vi "borders and shading constant (table).vi"() -> (0 "borders and shading":T1={"OutsideLineStyle"=1, "OutsideColor"=-16777216, "OutsideLineWidth"=2, "InsideLineStyle"=1, "InsideColor"=-16777216, "InsideLineWidth"=2, "BackgroundPatternColor"=-16777216} {"InsideLineStyle" items=["wdLineStyleNone", "wdLineStyleSingle", "wdLineStyleDot", "wdLineStyleDashSmallGap", "wdLineStyleDashLargeGap", "wdLineStyleDashDot", "wdLineStyleDashDotDot", "wdLineStyleDouble", "wdLineStyleTriple", "wdLineStyleThinThickSmallGap", "wdLineStyleThickThinSmallGap", "wdLineStyleThinThickThinSmallGap", "wdLineStyleThinThickMedGap", "wdLineStyleThickThinMedGap", "wdLineStyleThinThickThinMedGap", "wdLineStyleThinThickLargeGap", "wdLineStyleThickThinLargeGap", "wdLineStyleThinThickThinLargeGap", "wdLineStyleSingleWavy", "wdLineStyleDoubleWavy", "wdLineStyleDashDotStroked", "wdLineStyleEmboss3D", "wdLineStyleEngrave3D", "wdLineStyleOutset", "wdLineStyleInset"]; "BackgroundPatternColor" items=["wdColorAutomatic"=-16777216, "wdColorBlack"=0, "wdColorBlue"=16711680, "wdColorTurquoise"=16776960, "wdColorBrightGreen"=65280, "wdColorPink"=16711935, "wdColorRed"=255, "wdColorYellow"=65535, "wdColorWhite"=16777215, "wdColorDarkBlue"=8388608, "wdColorTeal"=8421376, "wdColorGreen"=32768, "wdColorViolet"=8388736, "wdColorDarkRed"=128, "wdColorDarkYellow"=32896, "wdColorBrown"=13209, "wdColorOliveGreen"=13107, "wdColorDarkGreen"=13056, "wdColorDarkTeal"=6697728, "wdColorIndigo"=10040115, "wdColorOrange"=26367, "wdColorBlueGray"=10053222, "wdColorLightOrange"=39423, "wdColorLime"=52377, "wdColorSeaGreen"=6723891, "wdColorAqua"=13421619, "wdColorLightBlue"=16737843, "wdColorGold"=52479, "wdColorSkyBlue"=16763904, "wdColorPlum"=6697881, "wdColorRose"=13408767, "wdColorTan"=10079487, "wdColorLightYellow"=10092543, "wdColorLightGreen"=13434828, "wdColorLightTurquoise"=16777164, "wdColorPaleBlue"=16764057, "wdColorLavender"=16751052, "wdColorGray05"=15987699, "wdColorGray10"=15132390, "wdColorGray125"=14737632, "wdColorGray15"=14277081, "wdColorGray20"=13421772, "wdColorGray25"=12632256, "wdColorGray30"=11776947, "wdColorGray35"=10921638, "wdColorGray375"=10526880, "wdColorGray40"=10066329, "wdColorGray45"=9211020, "wdColorGray50"=8421504, "wdColorGray55"=7566195, "wdColorGray60"=6710886, "wdColorGray625"=6316128, "wdColorGray65"=5855577, "wdColorGray70"=5000268, "wdColorGray75"=4210752, "wdColorGray80"=3355443, "wdColorGray85"=2500134, "wdColorGray875"=2105376, "wdColorGray90"=1644825, "wdColorGray95"=789516]; "InsideLineWidth" items=["wdLineWidth025pt"=2, "wdLineWidth050pt"=4, "wdLineWidth075pt"=6, "wdLineWidth100pt"=8, "wdLineWidth150pt"=12, "wdLineWidth225pt"=18, "wdLineWidth300pt"=24, "wdLineWidth450pt"=36, "wdLineWidth600pt"=48]; "InsideColor" items=["wdColorAutomatic"=-16777216, "wdColorBlack"=0, "wdColorBlue"=16711680, "wdColorTurquoise"=16776960, "wdColorBrightGreen"=65280, "wdColorPink"=16711935, "wdColorRed"=255, "wdColorYellow"=65535, "wdColorWhite"=16777215, "wdColorDarkBlue"=8388608, "wdColorTeal"=8421376, "wdColorGreen"=32768, "wdColorViolet"=8388736, "wdColorDarkRed"=128, "wdColorDarkYellow"=32896, "wdColorBrown"=13209, "wdColorOliveGreen"=13107, "wdColorDarkGreen"=13056, "wdColorDarkTeal"=6697728, "wdColorIndigo"=10040115, "wdColorOrange"=26367, "wdColorBlueGray"=10053222, "wdColorLightOrange"=39423, "wdColorLime"=52377, "wdColorSeaGreen"=6723891, "wdColorAqua"=13421619, "wdColorLightBlue"=16737843, "wdColorGold"=52479, "wdColorSkyBlue"=16763904, "wdColorPlum"=6697881, "wdColorRose"=13408767, "wdColorTan"=10079487, "wdColorLightYellow"=10092543, "wdColorLightGreen"=13434828, "wdColorLightTurquoise"=16777164, "wdColorPaleBlue"=16764057, "wdColorLavender"=16751052, "wdColorGray05"=15987699, "wdColorGray10"=15132390, "wdColorGray125"=14737632, "wdColorGray15"=14277081, "wdColorGray20"=13421772, "wdColorGray25"=12632256, "wdColorGray30"=11776947, "wdColorGray35"=10921638, "wdColorGray375"=10526880, "wdColorGray40"=10066329, "wdColorGray45"=9211020, "wdColorGray50"=8421504, "wdColorGray55"=7566195, "wdColorGray60"=6710886, "wdColorGray625"=6316128, "wdColorGray65"=5855577, "wdColorGray70"=5000268, "wdColorGray75"=4210752, "wdColorGray80"=3355443, "wdColorGray85"=2500134, "wdColorGray875"=2105376, "wdColorGray90"=1644825, "wdColorGray95"=789516]; "OutsideLineWidth" items=["wdLineWidth025pt"=2, "wdLineWidth050pt"=4, "wdLineWidth075pt"=6, "wdLineWidth100pt"=8, "wdLineWidth150pt"=12, "wdLineWidth225pt"=18, "wdLineWidth300pt"=24, "wdLineWidth450pt"=36, "wdLineWidth600pt"=48]; "OutsideColor" items=["wdColorAutomatic"=-16777216, "wdColorBlack"=0, "wdColorBlue"=16711680, "wdColorTurquoise"=16776960, "wdColorBrightGreen"=65280, "wdColorPink"=16711935, "wdColorRed"=255, "wdColorYellow"=65535, "wdColorWhite"=16777215, "wdColorDarkBlue"=8388608, "wdColorTeal"=8421376, "wdColorGreen"=32768, "wdColorViolet"=8388736, "wdColorDarkRed"=128, "wdColorDarkYellow"=32896, "wdColorBrown"=13209, "wdColorOliveGreen"=13107, "wdColorDarkGreen"=13056, "wdColorDarkTeal"=6697728, "wdColorIndigo"=10040115, "wdColorOrange"=26367, "wdColorBlueGray"=10053222, "wdColorLightOrange"=39423, "wdColorLime"=52377, "wdColorSeaGreen"=6723891, "wdColorAqua"=13421619, "wdColorLightBlue"=16737843, "wdColorGold"=52479, "wdColorSkyBlue"=16763904, "wdColorPlum"=6697881, "wdColorRose"=13408767, "wdColorTan"=10079487, "wdColorLightYellow"=10092543, "wdColorLightGreen"=13434828, "wdColorLightTurquoise"=16777164, "wdColorPaleBlue"=16764057, "wdColorLavender"=16751052, "wdColorGray05"=15987699, "wdColorGray10"=15132390, "wdColorGray125"=14737632, "wdColorGray15"=14277081, "wdColorGray20"=13421772, "wdColorGray25"=12632256, "wdColorGray30"=11776947, "wdColorGray35"=10921638, "wdColorGray375"=10526880, "wdColorGray40"=10066329, "wdColorGray45"=9211020, "wdColorGray50"=8421504, "wdColorGray55"=7566195, "wdColorGray60"=6710886, "wdColorGray625"=6316128, "wdColorGray65"=5855577, "wdColorGray70"=5000268, "wdColorGray75"=4210752, "wdColorGray80"=3355443, "wdColorGray85"=2500134, "wdColorGray875"=2105376, "wdColorGray90"=1644825, "wdColorGray95"=789516]; "OutsideLineStyle" items=["wdLineStyleNone", "wdLineStyleSingle", "wdLineStyleDot", "wdLineStyleDashSmallGap", "wdLineStyleDashLargeGap", "wdLineStyleDashDot", "wdLineStyleDashDotDot", "wdLineStyleDouble", "wdLineStyleTriple", "wdLineStyleThinThickSmallGap", "wdLineStyleThickThinSmallGap", "wdLineStyleThinThickThinSmallGap", "wdLineStyleThinThickMedGap", "wdLineStyleThickThinMedGap", "wdLineStyleThinThickThinMedGap", "wdLineStyleThinThickLargeGap", "wdLineStyleThickThinLargeGap", "wdLineStyleThinThickThinLargeGap", "wdLineStyleSingleWavy", "wdLineStyleDoubleWavy", "wdLineStyleDashDotStroked", "wdLineStyleEmboss3D", "wdLineStyleEngrave3D", "wdLineStyleOutset", "wdLineStyleInset"]})   [LabVIEW 2020, in "NI_ReportGenerationToolkit.lvlib"]
doc: "Defines the borders and shading attributes of a table in Word."
uses:
  <vilib>/addons/_office/NI_ReportGenerationToolkit.lvlib
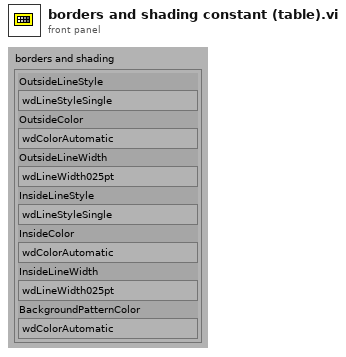
[diagram p1: front panel]
types:
  T1 = cluster{"OutsideLineStyle":i32, "OutsideColor":i32, "OutsideLineWidth":i32, "InsideLineStyle":i32, "InsideColor":i32, "InsideLineWidth":i32, "BackgroundPatternColor":i32}
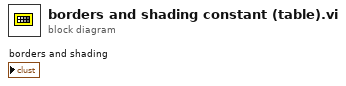
[diagram p0: block diagram]
diagram:
